vi "SmartSEM Remote API FIB Faraday cup.vi"(8 "error in":errorcluster, 11 "Api":refnum<k7>(container)) -> (0 "error out":errorcluster, 2 "FIB Faraday Cup (nA)":sgl, 3 "Api out":refnum<k7>)   [LabVIEW 2018]
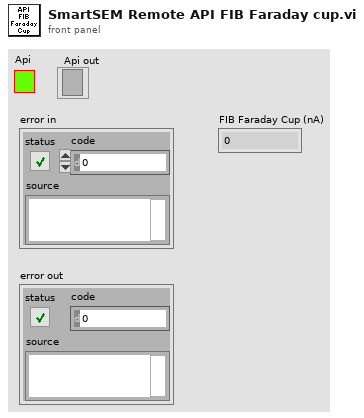
[diagram p1: front panel]
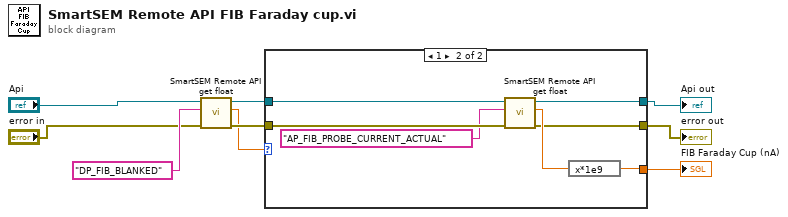
[diagram p0: block diagram]
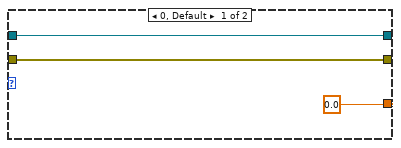
[diagram p2: hidden frame]
diagram:
  n1 = call "SmartSEM Remote API get float.vi"("error in"="error in", "lpszParam"="DP_FIB_BLANKED", "Api"="Api") -> ("error out"=w2:errorcluster, "vValue"=w1:sgl, "Api out"=w3:refnum<k7>)  [unwired: 6 in]
  n2 = case shown="1" w1 {
    tunnel: w3 -> [w12 w18]
    tunnel: w2 -> [w11 w17]
    tunnel: [w12 w14] -> w9
    tunnel: [w11 w13] -> w8
    tunnel: [sgl 0.0 w19] -> w7
    frame 0, Default {
    }
    frame 1 {
      n3 = call "SmartSEM Remote API get float.vi"("error in"=w17, "lpszParam"="AP_FIB_PROBE_CURRENT_ACTUAL", "Api"=w18) -> ("error out"=w13:errorcluster, "vValue"=w15:sgl, "Api out"=w14:refnum<k7>)  [unwired: 6 in]
      n4 = expression code="x*1e9"(w15) -> (w19:sgl)
    }
  }
  "Api out" <- w9
  "error out" <- w8
  "FIB Faraday Cup (nA)" <- w7
